vi "Rename And Move Entire Library By Name.vi"(8 "error in (no error)":errorcluster, 9 "Delete old directory if empty after move? (T)":bool=TRUE, 10 "New name without file extension":string, 11 "Library ref in":refnum<vi>) -> (0 "error out":errorcluster, 2 "New Library Path":path, 3 "Library ref out":refnum<vi>)   [LabVIEW 2020, in "Edit LVLibs.lvlib"]
doc: "Given a new name for this library, this VI will move that VI to a new directory next to the directory the library is currently in. The new directory will be named the same as the library minus the file extension. Then all the member VIs and sublibraries of the library will also be moved to the new directory maintaining their relative positions. Any member of the library that was not in the same directory as the library or a sublibrary will not be moved at all. By default, the old directory will be deleted after the move if it is empty of all files. The library and all members of the library will be saved at the end of this move to ensure that all files stay in sync with each other. Other files in memory that reference the library or its members will be modified to point to the new location but will not be saved."
uses:
  <vilib>/Utility/EditLVLibs/Edit LVLibs.lvlib
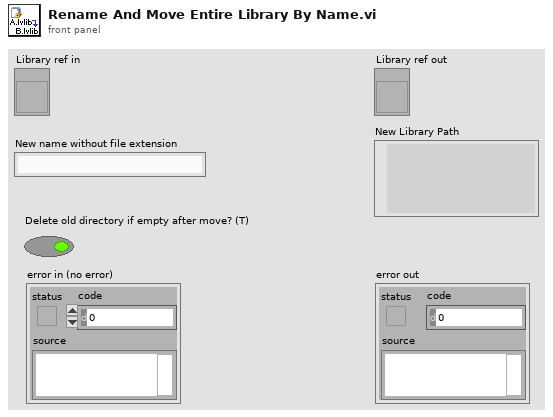
[diagram p1: front panel]
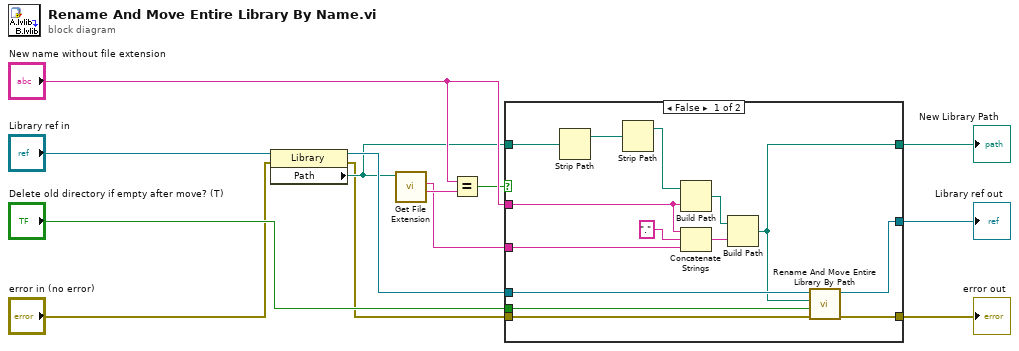
[diagram p0: block diagram]
diagram:
  n1 = property class="Library"(reference="Library ref in", error in="error in (no error)") -> (reference out=w8:refnum<vi>, error out=w1:errorcluster, "Path"=w6:path)
  n2 = call <vilib>:"Get File Extension.vi"("file"=w6) -> ("filename without extension"=w5:string, "lowercase file extension"=w4:string)  [unwired: 6 in, 3 out]
  n3 = Equal?(x="New name without file extension", y=w5) -> (x = y?=w11:bool)
  n4 = case shown="False" w11 {
    tunnel: "New name without file extension" -> [w23 _]
    tunnel: [w27 w30] -> w13
    tunnel: w1 -> [w18 w30]
    tunnel: [w21 w29] -> w10
    tunnel: w8 -> [w20 w29]
    tunnel: "Delete old directory if empty after move? (T)" -> [w19 _]
    tunnel: w6 -> [w16 w28]
    tunnel: w4 -> [w15 _]
    tunnel: [w14 w28] -> w3
    frame False {
      n5 = Strip Path(path=w16) -> (stripped path=w17:path)  [unwired: 1 out]
      n6 = Strip Path(path=w17) -> (stripped path=w26:path)  [unwired: 1 out]
      n7 = Build Path(base path=w26, name or relative path=w23) -> (appended path=w25:path)
      n8 = Concatenate Strings(w23, "." ("string"), w15) -> (w22:string)
      n9 = Build Path(base path=w25, name or relative path=w22) -> (appended path=w14:path)
      n10 = call <vilib>:"Rename And Move Entire Library By Path.vi"("error in (no error)"=w18, "Delete old directory if empty after move? (T)"=w19, "New library path"=w14, "Library ref in"=w20) -> ("error out"=w27:errorcluster, "Library ref out"=w21:refnum<vi>)  [unwired: 6 in]
    }
    frame True {
    }
  }
  "error out" <- w13
  "Library ref out" <- w10
  "New Library Path" <- w3
